vi "NISE.Log In.vi"(0 "SLSC Interface in":refnum<class "SLSC Interface.lvclass">, 1 "username":string, 2 "password":string, 5 "chassis":refnum<k21>, 11 "error in (no error)":errorcluster, 12 "connect timeout (60 sec)":dbl=60.0, 13 "save credentials to disk? (F)":bool) -> (4 "SLSC Interface out":refnum<class "SLSC Interface.lvclass">, 15 "error out":errorcluster)   [LabVIEW 2016, in "SLSC Interface.lvclass"]
uses:
  SLSC Interface.lvclass
  SLSC Interface.lvclass/SLSC Interface.ctl
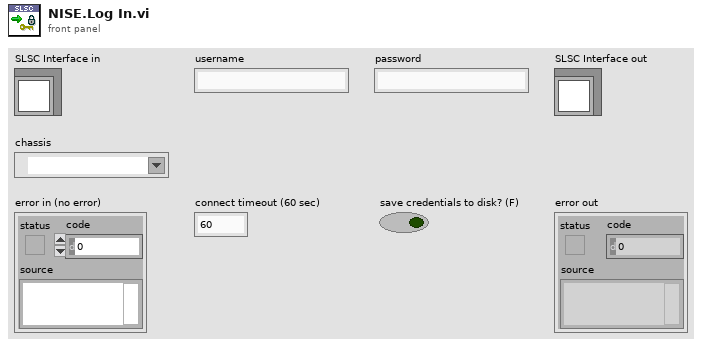
[diagram p1: front panel]
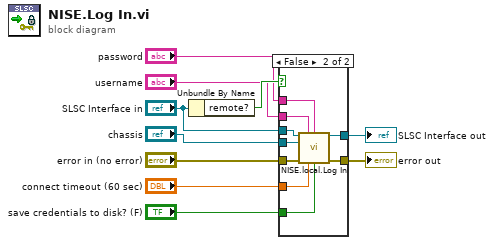
[diagram p0: block diagram]
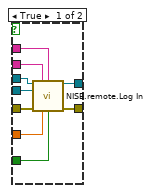
[diagram p2: hidden frame]
diagram:
  n1 = Unbundle By Name("SLSC Interface in") -> ("remote?"=w10:bool)
  n2 = case shown="False" w10 {
    tunnel: "SLSC Interface in" -> [w19 w28]
    tunnel: "username" -> [w18 w27]
    tunnel: "password" -> [w17 w26]
    tunnel: [w16 w25] -> w7
    tunnel: "chassis" -> [w15 w24]
    tunnel: "error in (no error)" -> [w14 w23]
    tunnel: "connect timeout (60 sec)" -> [w13 w22]
    tunnel: "save credentials to disk? (F)" -> [w12 w21]
    tunnel: [w11 w20] -> w2
    frame True {
      n3 = call "NISE.remote.Log In.vi"("SLSC Remote in"=w19, "username"=w18, "password"=w17, "chassis"=w15, "error in (no error)"=w14, "connect timeout (60 sec)"=w13, "save credentials to disk? (F)"=w12) -> ("SLSC Remote out"=w16:refnum<class "SLSC Interface.lvclass">, "error out"=w11:errorcluster)  [unwired: 7 in]
    }
    frame False {
      n4 = call "NISE.local.Log In.vi"("SLSC Local in"=w28, "username"=w27, "password"=w26, "chassis"=w24, "error in (no error)"=w23, "connect timeout (60 sec)"=w22, "save credentials to disk? (F)"=w21) -> ("SLSC Local out"=w25:refnum<class "SLSC Interface.lvclass">, "error out"=w20:errorcluster)  [unwired: 7 in]
    }
  }
  "error out" <- w2
  "SLSC Interface out" <- w7
